vi "test5-AsyncMessageWithReply.vi"(8 "error in (no error)":errorcluster, 11 "TestCase in":refnum<class "testcase-CSMMessage.lvclass">) -> (0 "error out":errorcluster, 3 "TestCase out":refnum<class "testcase-CSMMessage.lvclass">)   [LabVIEW 2017, in "testcase-CSMMessage.lvclass"]
uses:
  testcase-CSMMessage.lvclass
  7412589e-de49-4983-aece-358686b48526.vi
  src/user.lib/_NEVSTOP/Communicable State Machine(CSM)/AdvanceAPI/CSM - Make String Arguments Safe.vi
  src/user.lib/_NEVSTOP/Communicable State Machine(CSM)/AdvanceAPI/CSM - Keywords.vi
  <vilib>/addons/_JKI Toolkits/VI Tester/TestCase.llb/TestCase.lvclass
  src/user.lib/_NEVSTOP/Communicable State Machine(CSM)/Communicable State Machine.lvlib
  C:/Program Files (x86)/National Instruments/LabVIEW 2017/vi.lib/addons/_JKI Toolkits/VI Tester/TestCase.llb/TestCase.lvclass
panel:
  out "Loop count":i32
  out "concatenated string":string
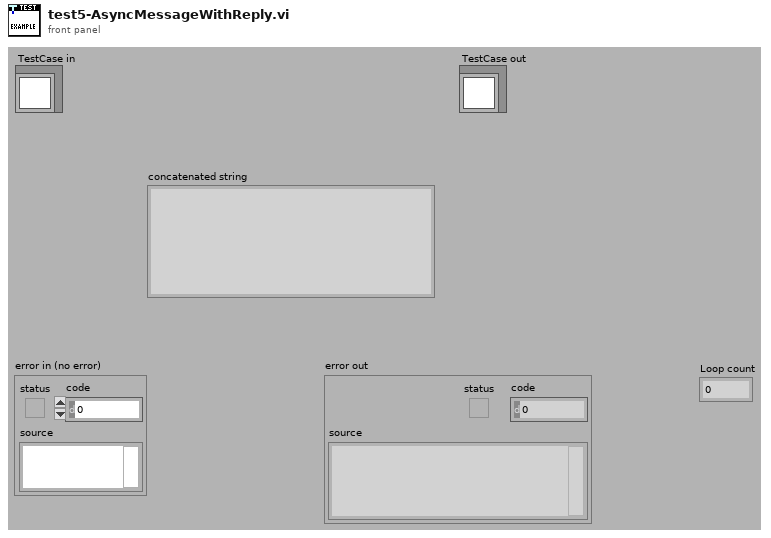
[diagram p1: front panel]
types:
  T1 = cluster{"Arguments":string, "Response":string, "error":errorcluster}
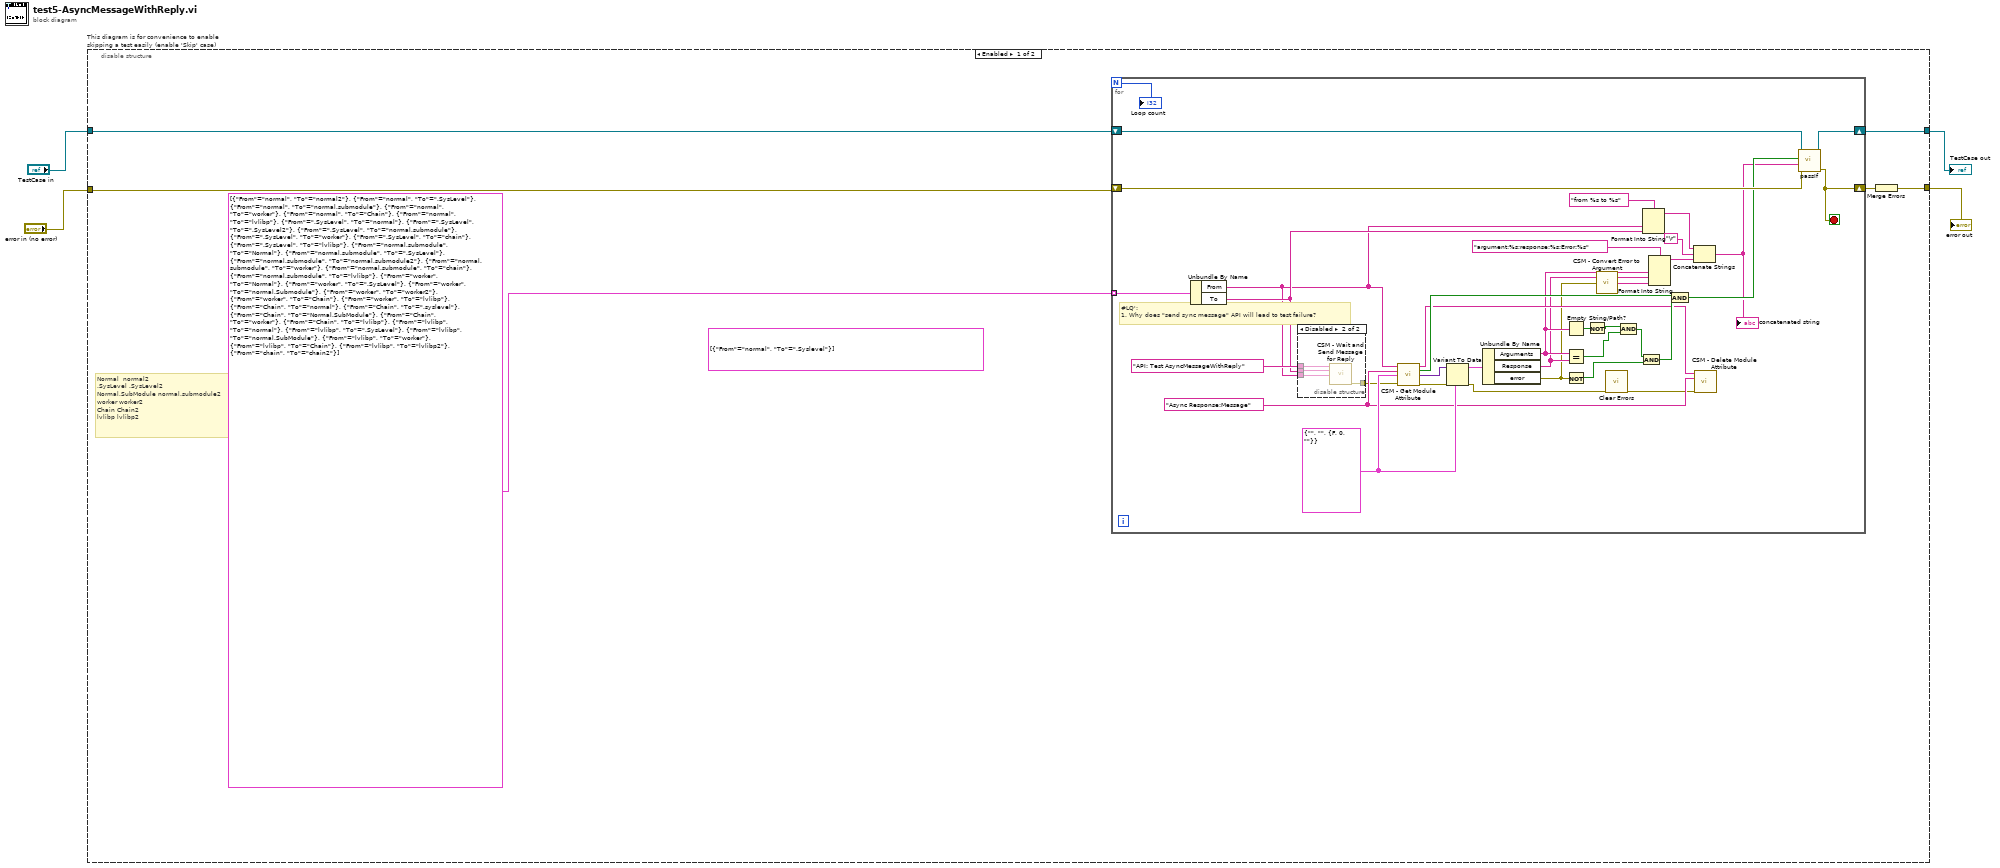
[diagram p0: block diagram]
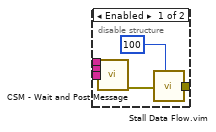
[diagram p2: hidden frame]
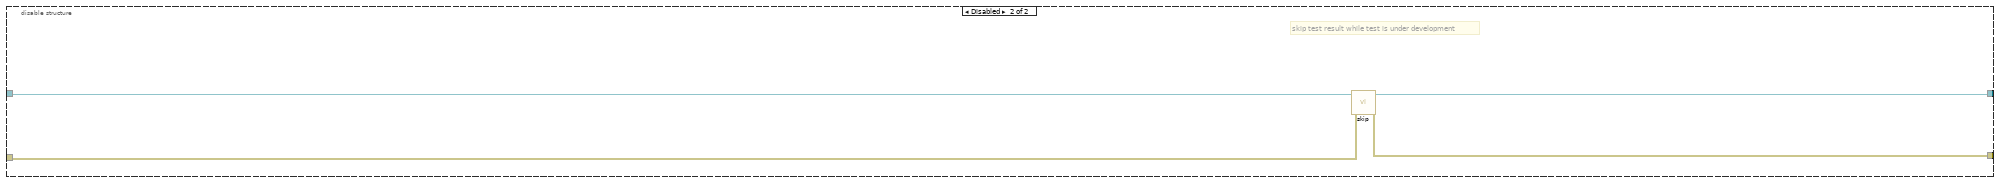
[diagram p3: hidden frame]
diagram:
  n1 = disable-structure "This diagram is for convenience to enable skipping a test easily (enable 'Skip' case)" shown="Enabled" {
    disable-tunnel: "TestCase in" -> [w10 w60]
    disable-tunnel: [w9 w58] -> w1
    disable-tunnel: [w6 w59] -> w3
    disable-tunnel: "error in (no error)" -> [w7 w57]
    frame Enabled {
      (unwired) cluster{"From":string, "To":string}[] [{"From"="normal", "To"=".Syslevel"}]
      # "Normal  normal2\n.SysLevel .SysLevel2\nNormal.SubModule normal.submodule2\nworker worker2\nChain Chain2\nlvlibp lvlibp2"
      n2 = for {
        N -> [w11]
        tunnel: cluster{"From":string, "To":string}[] [{"From"="normal", "To"="normal2"}, {"From"="normal", "To"=".SysLevel"}, {"From"="normal", "To"="normal.submodule"}, {"From"="normal", "To"="worker"}, {"From"="normal", "To"="Chain"}, {"From"="normal", "To"="lvlibp"}, {"From"=".SysLevel", "To"="normal"}, {"From"=".SysLevel", "To"=".SysLevel2"}, {"From"=".SysLevel", "To"="normal.submodule"}, {"From"=".SysLevel", "To"="worker"}, {"From"=".SysLevel", "To"="chain"}, {"From"=".SysLevel", "To"="lvlibp"}, {"From"="normal.submodule", "To"="Normal"}, {"From"="normal.submodule", "To"=".SysLevel"}, {"From"="normal.submodule", "To"="normal.submodule2"}, {"From"="normal.submodule", "To"="worker"}, {"From"="normal.submodule", "To"="chain"}, {"From"="normal.submodule", "To"="lvlibp"}, {"From"="worker", "To"="Normal"}, {"From"="worker", "To"=".SysLevel"}, {"From"="worker", "To"="normal.Submodule"}, {"From"="worker", "To"="worker2"}, {"From"="worker", "To"="Chain"}, {"From"="worker", "To"="lvlibp"}, {"From"="Chain", "To"="normal"}, {"From"="Chain", "To"=".syslevel"}, {"From"="Chain", "To"="Normal.SubModule"}, {"From"="Chain", "To"="worker"}, {"From"="Chain", "To"="lvlibp"}, {"From"="lvlibp", "To"="normal"}, {"From"="lvlibp", "To"=".SysLevel"}, {"From"="lvlibp", "To"="normal.SubModule"}, {"From"="lvlibp", "To"="worker"}, {"From"="lvlibp", "To"="Chain"}, {"From"="lvlibp", "To"="lvlibp2"}, {"From"="chain", "To"="chain2"}] -> [w34] mode=indexing
        shift-right: [w45] -> w9
        shift-left: w10 -> [w46]
        shift-right: [w14] -> w8
        shift-left: w7 -> [w44]
        stop <- w14 stop-if-true
        w41 = T1 {"Arguments"="", "Response"="", "error"={"status"=FALSE, "code"=0, "source"=""}}
        w30 = "Async Response:Message" ("State")
        # "#LQ':\n1. Why does \"send sync message\" API will lead to test failure?"
        n3 = Unbundle By Name(w34) -> ("From"=w13:string, "To"=w33:string)
        n4 = disable-structure shown="Disabled" {
          disable-tunnel: "API: Test AsyncMessageWithReply" ("State") -> [w52 w55]
          disable-tunnel: w33 -> [w51 w54]
          disable-tunnel: w13 -> [w50 w53]
          disable-tunnel: [w48 w56] -> w12
          frame Enabled {
            n5 = call "CSM - Wait and Post Message.vi"("State"=w52, "Arguments (\"\")"=w51, "Target Module"=w50) -> ("error out"=w49:errorcluster)  [unwired: 12 in]
            n6 = call "Stall Data Flow.vim"("value in"=w49, "milliseconds to wait"=u32 100) -> ("value out"=w48:errorcluster)  [unwired: 1 out]
          }
          frame Disabled {
            n7 = call "CSM - Wait and Send Message for Reply.vi"("State"=w55, "Arguments (\"\")"=w54, "Target Module"=w53) -> ("error out"=w56:errorcluster)  [unwired: 10 in, 2 out]
          }
        }
        n8 = call "CSM - Get Module Attribute.vi"("CSM Name"=w13, "Attribute"=w30, "Default Value (Empty Variant)"=w41, "Error In"=w12) -> ("CSM Name (Dup)"=w31:string, "Found"=w37:bool, "Value"=w40:variant, "error out"=w42:errorcluster)  [unwired: 7 in, 1 out]
        n9 = Variant To Data(error in=w42, type=w41, Variant=w40) -> (data=w39:T1, error out=w16:errorcluster)
        n10 = Unbundle By Name(w39) -> ("Arguments"=w25:string, "Response"=w24:string, "error"=w22:errorcluster)
        n11 = Empty String/Path?(string/path=w25) -> (empty?=w29:bool)
        n12 = Equal?(x=w25, y=w24) -> (x = y?=w27:bool)
        n13 = Not(x=w22) -> (.not. x?=w38:bool)
        n14 = Not(x=w29) -> (.not. x?=w28:bool)
        n15 = call "CSM - Convert Error to Argument.vi"("Error"=w22) -> ("Argument"=w23:string)  [unwired: 4 in]
        n16 = call <vilib>:"Clear Errors.vi"("error in (no error)"=w16) -> ("error out"=w15:errorcluster)  [unwired: 5 in, 1 out]
        n17 = And(x=w28, y=w27) -> (x .and. y?=w26:bool)
        n18 = And(x=w26, y=w38) -> (x .and. y?=w36:bool)
        n19 = Format Into String(format string="from %s to %s", w13, w33) -> (resulting string=w18:string)  [unwired: 2 in, 1 out]
        n20 = Format Into String(format string="argument:%s;response:%s;Error:%s", w25, w24, w23) -> (resulting string=w21:string)  [unwired: 2 in, 1 out]
        n21 = And(x=w37, y=w36) -> (x .and. y?=w35:bool)
        n22 = Concatenate Strings(w18, "\r", w21) -> (w19:string)
        "concatenated string" <- w19
        n23 = call "CSM - Delete Module Attribute.vi"("CSM Name"=w31, "Attribute"=w30, "Error In"=w15) -> ()  [unwired: 9 in, 4 out]
        n24 = call-dynamic "passIf.vi"("error in (no error)"=w44, "message (\"\")"=w19, "pass"=w35, "TestCase in"=w46) -> ("error out"=w14:errorcluster, "TestCase out"=w45:refnum<class "testcase-CSMMessage.lvclass">)  [unwired: 6 in]
        "Loop count" <- w11
      }
      n25 = Merge Errors(w8) -> (w6:errorcluster)
    }
    frame Disabled {
      # "skip test result while test is under development"
      n26 = call <vilib>:"skip.vi"("error in (no error)"=w57, "TestCase in"=w60) -> ("error out"=w59:errorcluster, "TestCase out"=w58:refnum<class "testcase-CSMMessage.lvclass">)  [unwired: 8 in]
    }
  }
  "error out" <- w3
  "TestCase out" <- w1
